vi "Zluta-Rolnicky.vi"(11 "NXT/EV3":T1) -> (3 "NXT/EV3 2":T1)   [LabVIEW 2016]
uses:
  <vilib>/NXT/Subs/LVHSConnector.ctl
  <vilib>/NXT/LegoClasses/BrickReference/BrickReference.lvclass
  <vilib>/NXT/Dual Mode Library/Display/drawText_Center.vi
  <vilib>/NXT/Dual Mode Library/Sound/PlayD.vi
  <vilib>/NXT/Dual Mode Library/Sound/PlayB.vi
  <vilib>/NXT/Dual Mode Library/Sound/PlayA.vi
  <vilib>/NXT/Dual Mode Library/Sound/PlayG.vi
  <vilib>/NXT/Dual Mode Library/Sound/PlayE.vi
  <vilib>/NXT/Dual Mode Library/Sound/PlayC.vi
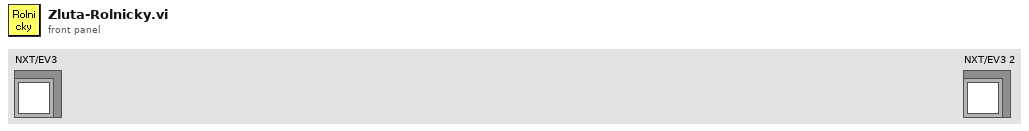
[diagram p1: front panel]
types:
  T1 = typedef "LVHSConnector.ctl" = refnum<class "BrickReference.lvclass">
diagram:
  w13 = u16 4 items=["3"=3, "4"=4, "5"=5, "6"=6, "7"=7] ("Octave")
  w14 = u16 4 items=["3"=3, "4"=4, "5"=5, "6"=6, "7"=7] ("Octave")
  w10 = u16 5 items=["3"=3, "4"=4, "5"=5, "6"=6, "7"=7] ("Octave")
  w5 = u16 5 items=["3"=3, "4"=4, "5"=5, "6"=6, "7"=7] ("Octave")
  w4 = u16 5 items=["3"=3, "4"=4, "5"=5, "6"=6, "7"=7] ("Octave")
  w20 = u16 4 items=["3"=3, "4"=4, "5"=5, "6"=6, "7"=7] ("Octave")
  w23 = u16 4 items=["3"=3, "4"=4, "5"=5, "6"=6, "7"=7] ("Octave")
  w28 = u16 4 items=["3"=3, "4"=4, "5"=5, "6"=6, "7"=7] ("Octave")
  w29 = u16 5 items=["3"=3, "4"=4, "5"=5, "6"=6, "7"=7] ("Octave")
  w38 = u16 5 items=["3"=3, "4"=4, "5"=5, "6"=6, "7"=7] ("Octave")
  w33 = u16 5 items=["3"=3, "4"=4, "5"=5, "6"=6, "7"=7] ("Octave")
  w32 = u16 5 items=["3"=3, "4"=4, "5"=5, "6"=6, "7"=7] ("Octave")
  w43 = u16 4 items=["3"=3, "4"=4, "5"=5, "6"=6, "7"=7] ("Octave")
  w44 = u16 4 items=["3"=3, "4"=4, "5"=5, "6"=6, "7"=7] ("Octave")
  w47 = u16 4 items=["3"=3, "4"=4, "5"=5, "6"=6, "7"=7] ("Octave")
  w50 = u16 5 items=["3"=3, "4"=4, "5"=5, "6"=6, "7"=7] ("Octave")
  w53 = u16 4 items=["3"=3, "4"=4, "5"=5, "6"=6, "7"=7] ("Octave")
  w62 = u16 4 items=["3"=3, "4"=4, "5"=5, "6"=6, "7"=7] ("Octave")
  w57 = u16 4 items=["3"=3, "4"=4, "5"=5, "6"=6, "7"=7] ("Octave")
  w56 = u16 4 items=["3"=3, "4"=4, "5"=5, "6"=6, "7"=7] ("Octave")
  w63 = u16 4 items=["3"=3, "4"=4, "5"=5, "6"=6, "7"=7] ("Octave")
  w68 = u16 4 items=["3"=3, "4"=4, "5"=5, "6"=6, "7"=7] ("Octave")
  w69 = u16 4 items=["3"=3, "4"=4, "5"=5, "6"=6, "7"=7] ("Octave")
  w73 = u16 5 items=["3"=3, "4"=4, "5"=5, "6"=6, "7"=7] ("Octave")
  w74 = u16 4 items=["3"=3, "4"=4, "5"=5, "6"=6, "7"=7] ("Octave")
  w78 = u16 4 items=["3"=3, "4"=4, "5"=5, "6"=6, "7"=7] ("Octave")
  w82 = u16 4 items=["3"=3, "4"=4, "5"=5, "6"=6, "7"=7] ("Octave")
  w84 = u16 4 items=["3"=3, "4"=4, "5"=5, "6"=6, "7"=7] ("Octave")
  w86 = u16 4 items=["3"=3, "4"=4, "5"=5, "6"=6, "7"=7] ("Octave")
  w91 = u16 4 items=["3"=3, "4"=4, "5"=5, "6"=6, "7"=7] ("Octave")
  w96 = u16 4 items=["3"=3, "4"=4, "5"=5, "6"=6, "7"=7] ("Octave")
  w97 = u16 5 items=["3"=3, "4"=4, "5"=5, "6"=6, "7"=7] ("Octave")
  w106 = u16 5 items=["3"=3, "4"=4, "5"=5, "6"=6, "7"=7] ("Octave")
  w101 = u16 5 items=["3"=3, "4"=4, "5"=5, "6"=6, "7"=7] ("Octave")
  w100 = u16 5 items=["3"=3, "4"=4, "5"=5, "6"=6, "7"=7] ("Octave")
  w112 = u16 4 items=["3"=3, "4"=4, "5"=5, "6"=6, "7"=7] ("Octave")
  w113 = u16 4 items=["3"=3, "4"=4, "5"=5, "6"=6, "7"=7] ("Octave")
  w116 = u16 4 items=["3"=3, "4"=4, "5"=5, "6"=6, "7"=7] ("Octave")
  w119 = u16 5 items=["3"=3, "4"=4, "5"=5, "6"=6, "7"=7] ("Octave")
  w122 = u16 4 items=["3"=3, "4"=4, "5"=5, "6"=6, "7"=7] ("Octave")
  w131 = u16 4 items=["3"=3, "4"=4, "5"=5, "6"=6, "7"=7] ("Octave")
  w126 = u16 4 items=["3"=3, "4"=4, "5"=5, "6"=6, "7"=7] ("Octave")
  w125 = u16 4 items=["3"=3, "4"=4, "5"=5, "6"=6, "7"=7] ("Octave")
  w132 = u16 4 items=["3"=3, "4"=4, "5"=5, "6"=6, "7"=7] ("Octave")
  w137 = u16 4 items=["3"=3, "4"=4, "5"=5, "6"=6, "7"=7] ("Octave")
  w138 = u16 4 items=["3"=3, "4"=4, "5"=5, "6"=6, "7"=7] ("Octave")
  w196 = u16 4 items=["3"=3, "4"=4, "5"=5, "6"=6, "7"=7] ("Octave")
  w195 = u16 4 items=["3"=3, "4"=4, "5"=5, "6"=6, "7"=7] ("Octave")
  w194 = u16 5 items=["3"=3, "4"=4, "5"=5, "6"=6, "7"=7] ("Octave")
  w193 = u16 5 items=["3"=3, "4"=4, "5"=5, "6"=6, "7"=7] ("Octave")
  w192 = u16 5 items=["3"=3, "4"=4, "5"=5, "6"=6, "7"=7] ("Octave")
  w178 = u16 5 items=["3"=3, "4"=4, "5"=5, "6"=6, "7"=7] ("Octave")
  w175 = u16 5 items=["3"=3, "4"=4, "5"=5, "6"=6, "7"=7] ("Octave")
  w174 = u16 5 items=["3"=3, "4"=4, "5"=5, "6"=6, "7"=7] ("Octave")
  w173 = u16 5 items=["3"=3, "4"=4, "5"=5, "6"=6, "7"=7] ("Octave")
  w197 = u16 4 items=["3"=3, "4"=4, "5"=5, "6"=6, "7"=7] ("Octave")
  w198 = u16 4 items=["3"=3, "4"=4, "5"=5, "6"=6, "7"=7] ("Octave")
  w199 = u16 5 items=["3"=3, "4"=4, "5"=5, "6"=6, "7"=7] ("Octave")
  w200 = u16 5 items=["3"=3, "4"=4, "5"=5, "6"=6, "7"=7] ("Octave")
  w201 = u16 5 items=["3"=3, "4"=4, "5"=5, "6"=6, "7"=7] ("Octave")
  w215 = u16 5 items=["3"=3, "4"=4, "5"=5, "6"=6, "7"=7] ("Octave")
  w218 = u16 5 items=["3"=3, "4"=4, "5"=5, "6"=6, "7"=7] ("Octave")
  w219 = u16 5 items=["3"=3, "4"=4, "5"=5, "6"=6, "7"=7] ("Octave")
  w220 = u16 5 items=["3"=3, "4"=4, "5"=5, "6"=6, "7"=7] ("Octave")
  w255 = i16 0 items=["1", "2", "3", "4", "5", "6", "7", "8", "9", "10", "11", "12"] ("Line")
  n1 = call-poly <vilib>:"PolyDisplay.vi"("Text"="\n\n\n\n\nEV3 JUK3BOX:\nRolnicky \n\n\n\n\n\n\n\n\n\n", "NXT/EV3"="NXT/EV3", "Line"=w255) -> ("NXT/EV3"=w230:T1)  [unwired: 1 in]
  n2 = call-poly <vilib>:"PolySound.vi"("Duration (500 ms)"=u16 375, "NXT/EV3"=w230) -> ("NXT/EV3"=w251:T1)  [unwired: 2 in]
  n3 = call-poly <vilib>:"PolySound.vi"("Duration (500 ms)"=u16 375, "NXT/EV3"=w251) -> ("NXT/EV3"=w247:T1)  [unwired: 2 in]
  n4 = call-poly <vilib>:"PolySound.vi"("Duration (500 ms)"=u16 375, "NXT/EV3"=w247) -> ("NXT/EV3"=w246:T1)  [unwired: 2 in]
  n5 = call-poly <vilib>:"PolySound.vi"("Duration (500 ms)"=u16 375, "NXT/EV3"=w246) -> ("NXT/EV3"=w245:T1)  [unwired: 2 in]
  n6 = call-poly <vilib>:"PolySound.vi"("Duration (500 ms)"=u16 1125, "NXT/EV3"=w245) -> ("NXT/EV3"=w242:T1)  [unwired: 2 in]
  n7 = call-poly <vilib>:"PolySound.vi"("Duration (500 ms)"=u16 375, "NXT/EV3"=w242) -> ("NXT/EV3"=w241:T1)  [unwired: 2 in]
  n8 = call-poly <vilib>:"PolySound.vi"("Duration (500 ms)"=u16 375, "NXT/EV3"=w241) -> ("NXT/EV3"=w235:T1)  [unwired: 2 in]
  n9 = call-poly <vilib>:"PolySound.vi"("Duration (500 ms)"=u16 375, "NXT/EV3"=w235) -> ("NXT/EV3"=w236:T1)  [unwired: 2 in]
  n10 = call-poly <vilib>:"PolySound.vi"("Duration (500 ms)"=u16 375, "NXT/EV3"=w236) -> ("NXT/EV3"=w240:T1)  [unwired: 2 in]
  n11 = call-poly <vilib>:"PolySound.vi"("Duration (500 ms)"=u16 375, "NXT/EV3"=w240) -> ("NXT/EV3"=w231:T1)  [unwired: 2 in]
  n12 = call-poly <vilib>:"PolySound.vi"("Duration (500 ms)"=u16 1125, "NXT/EV3"=w231) -> ("NXT/EV3"=w234:T1)  [unwired: 2 in]
  n13 = call-poly <vilib>:"PolySound.vi"("Duration (500 ms)"=u16 375, "NXT/EV3"=w234) -> ("NXT/EV3"=w202:T1)  [unwired: 2 in]
  n14 = call-poly <vilib>:"PolySound.vi"("Duration (500 ms)"=u16 375, "NXT/EV3"=w202) -> ("NXT/EV3"=w223:T1)  [unwired: 2 in]
  n15 = call-poly <vilib>:"PolySound.vi"("Duration (500 ms)"=u16 375, "NXT/EV3"=w223, "Octave"=w220) -> ("NXT/EV3"=w227:T1)  [unwired: 1 in]
  n16 = call-poly <vilib>:"PolySound.vi"("Duration (500 ms)"=u16 375, "NXT/EV3"=w227) -> ("NXT/EV3"=w228:T1)  [unwired: 2 in]
  n17 = call-poly <vilib>:"PolySound.vi"("Duration (500 ms)"=u16 375, "NXT/EV3"=w228) -> ("NXT/EV3"=w229:T1)  [unwired: 2 in]
  n18 = call-poly <vilib>:"PolySound.vi"("Duration (500 ms)"=u16 375, "NXT/EV3"=w229, "Octave"=w219) -> ("NXT/EV3"=w214:T1)  [unwired: 1 in]
  n19 = call-poly <vilib>:"PolySound.vi"("Duration (500 ms)"=u16 375, "NXT/EV3"=w214, "Octave"=w218) -> ("NXT/EV3"=w213:T1)  [unwired: 1 in]
  n20 = call-poly <vilib>:"PolySound.vi"("Duration (500 ms)"=u16 750, "NXT/EV3"=w213, "Octave"=w215) -> ("NXT/EV3"=w207:T1)  [unwired: 1 in]
  n21 = call-poly <vilib>:"PolySound.vi"("Duration (500 ms)"=u16 375, "NXT/EV3"=w207, "Octave"=w201) -> ("NXT/EV3"=w206:T1)  [unwired: 1 in]
  n22 = call-poly <vilib>:"PolySound.vi"("Duration (500 ms)"=u16 375, "NXT/EV3"=w206, "Octave"=w200) -> ("NXT/EV3"=w205:T1)  [unwired: 1 in]
  n23 = call-poly <vilib>:"PolySound.vi"("Duration (500 ms)"=u16 375, "NXT/EV3"=w205, "Octave"=w199) -> ("NXT/EV3"=w204:T1)  [unwired: 1 in]
  n24 = call-poly <vilib>:"PolySound.vi"("Duration (500 ms)"=u16 375, "NXT/EV3"=w204, "Octave"=w198) -> ("NXT/EV3"=w203:T1)  [unwired: 1 in]
  n25 = call-poly <vilib>:"PolySound.vi"("Duration (500 ms)"=u16 1500, "NXT/EV3"=w203, "Octave"=w197) -> ("NXT/EV3"=w140:T1)  [unwired: 1 in]
  n26 = call-poly <vilib>:"PolySound.vi"("Duration (500 ms)"=u16 375, "NXT/EV3"=w140) -> ("NXT/EV3"=w143:T1)  [unwired: 2 in]
  n27 = call-poly <vilib>:"PolySound.vi"("Duration (500 ms)"=u16 375, "NXT/EV3"=w143) -> ("NXT/EV3"=w147:T1)  [unwired: 2 in]
  n28 = call-poly <vilib>:"PolySound.vi"("Duration (500 ms)"=u16 375, "NXT/EV3"=w147) -> ("NXT/EV3"=w148:T1)  [unwired: 2 in]
  n29 = call-poly <vilib>:"PolySound.vi"("Duration (500 ms)"=u16 375, "NXT/EV3"=w148) -> ("NXT/EV3"=w149:T1)  [unwired: 2 in]
  n30 = call-poly <vilib>:"PolySound.vi"("Duration (500 ms)"=u16 1125, "NXT/EV3"=w149) -> ("NXT/EV3"=w152:T1)  [unwired: 2 in]
  n31 = call-poly <vilib>:"PolySound.vi"("Duration (500 ms)"=u16 375, "NXT/EV3"=w152) -> ("NXT/EV3"=w153:T1)  [unwired: 2 in]
  n32 = call-poly <vilib>:"PolySound.vi"("Duration (500 ms)"=u16 375, "NXT/EV3"=w153) -> ("NXT/EV3"=w159:T1)  [unwired: 2 in]
  n33 = call-poly <vilib>:"PolySound.vi"("Duration (500 ms)"=u16 375, "NXT/EV3"=w159) -> ("NXT/EV3"=w158:T1)  [unwired: 2 in]
  n34 = call-poly <vilib>:"PolySound.vi"("Duration (500 ms)"=u16 375, "NXT/EV3"=w158) -> ("NXT/EV3"=w154:T1)  [unwired: 2 in]
  n35 = call-poly <vilib>:"PolySound.vi"("Duration (500 ms)"=u16 375, "NXT/EV3"=w154) -> ("NXT/EV3"=w163:T1)  [unwired: 2 in]
  n36 = call-poly <vilib>:"PolySound.vi"("Duration (500 ms)"=u16 1125, "NXT/EV3"=w163) -> ("NXT/EV3"=w160:T1)  [unwired: 2 in]
  n37 = call-poly <vilib>:"PolySound.vi"("Duration (500 ms)"=u16 375, "NXT/EV3"=w160) -> ("NXT/EV3"=w191:T1)  [unwired: 2 in]
  n38 = call-poly <vilib>:"PolySound.vi"("Duration (500 ms)"=u16 375, "NXT/EV3"=w191) -> ("NXT/EV3"=w170:T1)  [unwired: 2 in]
  n39 = call-poly <vilib>:"PolySound.vi"("Duration (500 ms)"=u16 375, "NXT/EV3"=w170, "Octave"=w173) -> ("NXT/EV3"=w166:T1)  [unwired: 1 in]
  n40 = call-poly <vilib>:"PolySound.vi"("Duration (500 ms)"=u16 375, "NXT/EV3"=w166) -> ("NXT/EV3"=w165:T1)  [unwired: 2 in]
  n41 = call-poly <vilib>:"PolySound.vi"("Duration (500 ms)"=u16 375, "NXT/EV3"=w165) -> ("NXT/EV3"=w164:T1)  [unwired: 2 in]
  n42 = call-poly <vilib>:"PolySound.vi"("Duration (500 ms)"=u16 375, "NXT/EV3"=w164, "Octave"=w174) -> ("NXT/EV3"=w179:T1)  [unwired: 1 in]
  n43 = call-poly <vilib>:"PolySound.vi"("Duration (500 ms)"=u16 375, "NXT/EV3"=w179, "Octave"=w175) -> ("NXT/EV3"=w180:T1)  [unwired: 1 in]
  n44 = call-poly <vilib>:"PolySound.vi"("Duration (500 ms)"=u16 750, "NXT/EV3"=w180, "Octave"=w178) -> ("NXT/EV3"=w186:T1)  [unwired: 1 in]
  n45 = call-poly <vilib>:"PolySound.vi"("Duration (500 ms)"=u16 375, "NXT/EV3"=w186, "Octave"=w192) -> ("NXT/EV3"=w187:T1)  [unwired: 1 in]
  n46 = call-poly <vilib>:"PolySound.vi"("Duration (500 ms)"=u16 375, "NXT/EV3"=w187, "Octave"=w193) -> ("NXT/EV3"=w188:T1)  [unwired: 1 in]
  n47 = call-poly <vilib>:"PolySound.vi"("Duration (500 ms)"=u16 375, "NXT/EV3"=w188, "Octave"=w194) -> ("NXT/EV3"=w189:T1)  [unwired: 1 in]
  n48 = call-poly <vilib>:"PolySound.vi"("Duration (500 ms)"=u16 375, "NXT/EV3"=w189, "Octave"=w195) -> ("NXT/EV3"=w190:T1)  [unwired: 1 in]
  n49 = call-poly <vilib>:"PolySound.vi"("Duration (500 ms)"=u16 1500, "NXT/EV3"=w190, "Octave"=w196) -> ("NXT/EV3"=w107:T1)  [unwired: 1 in]
  n50 = call-poly <vilib>:"PolySound.vi"("Duration (500 ms)"=u16 375, "NXT/EV3"=w107, "Octave"=w138) -> ("NXT/EV3"=w134:T1)  [unwired: 1 in]
  n51 = call-poly <vilib>:"PolySound.vi"("Duration (500 ms)"=u16 375, "NXT/EV3"=w134, "Octave"=w137) -> ("NXT/EV3"=w133:T1)  [unwired: 1 in]
  n52 = call-poly <vilib>:"PolySound.vi"("Duration (500 ms)"=u16 750, "NXT/EV3"=w133, "Octave"=w132) -> ("NXT/EV3"=w123:T1)  [unwired: 1 in]
  n53 = call-poly <vilib>:"PolySound.vi"("Duration (500 ms)"=u16 375, "NXT/EV3"=w123, "Octave"=w125) -> ("NXT/EV3"=w129:T1)  [unwired: 1 in]
  n54 = call-poly <vilib>:"PolySound.vi"("Duration (500 ms)"=u16 375, "NXT/EV3"=w129, "Octave"=w126) -> ("NXT/EV3"=w130:T1)  [unwired: 1 in]
  n55 = call-poly <vilib>:"PolySound.vi"("Duration (500 ms)"=u16 750, "NXT/EV3"=w130, "Octave"=w131) -> ("NXT/EV3"=w117:T1)  [unwired: 1 in]
  n56 = call-poly <vilib>:"PolySound.vi"("Duration (500 ms)"=u16 375, "NXT/EV3"=w117, "Octave"=w122) -> ("NXT/EV3"=w118:T1)  [unwired: 1 in]
  n57 = call-poly <vilib>:"PolySound.vi"("Duration (500 ms)"=u16 375, "NXT/EV3"=w118, "Octave"=w119) -> ("NXT/EV3"=w108:T1)  [unwired: 1 in]
  n58 = call-poly <vilib>:"PolySound.vi"("Duration (500 ms)"=u16 562, "NXT/EV3"=w108, "Octave"=w116) -> ("NXT/EV3"=w110:T1)  [unwired: 1 in]
  n59 = call-poly <vilib>:"PolySound.vi"("Duration (500 ms)"=u16 188, "NXT/EV3"=w110, "Octave"=w113) -> ("NXT/EV3"=w109:T1)  [unwired: 1 in]
  n60 = call-poly <vilib>:"PolySound.vi"("Duration (500 ms)"=u16 1500, "NXT/EV3"=w109, "Octave"=w112) -> ("NXT/EV3"=w89:T1)  [unwired: 1 in]
  n61 = call-poly <vilib>:"PolySound.vi"("Duration (500 ms)"=u16 375, "NXT/EV3"=w89, "Octave"=w100) -> ("NXT/EV3"=w104:T1)  [unwired: 1 in]
  n62 = call-poly <vilib>:"PolySound.vi"("Duration (500 ms)"=u16 375, "NXT/EV3"=w104, "Octave"=w101) -> ("NXT/EV3"=w105:T1)  [unwired: 1 in]
  n63 = call-poly <vilib>:"PolySound.vi"("Duration (500 ms)"=u16 750, "NXT/EV3"=w105, "Octave"=w106) -> ("NXT/EV3"=w90:T1)  [unwired: 1 in]
  n64 = call-poly <vilib>:"PolySound.vi"("Duration (500 ms)"=u16 375, "NXT/EV3"=w90, "Octave"=w97) -> ("NXT/EV3"=w93:T1)  [unwired: 1 in]
  n65 = call-poly <vilib>:"PolySound.vi"("Duration (500 ms)"=u16 375, "NXT/EV3"=w93, "Octave"=w96) -> ("NXT/EV3"=w92:T1)  [unwired: 1 in]
  n66 = call-poly <vilib>:"PolySound.vi"("Duration (500 ms)"=u16 750, "NXT/EV3"=w92, "Octave"=w91) -> ("NXT/EV3"=w83:T1)  [unwired: 1 in]
  n67 = call-poly <vilib>:"PolySound.vi"("Duration (500 ms)"=u16 375, "NXT/EV3"=w83, "Octave"=w86) -> ("NXT/EV3"=w88:T1)  [unwired: 1 in]
  n68 = call-poly <vilib>:"PolySound.vi"("Duration (500 ms)"=u16 375, "NXT/EV3"=w88, "Octave"=w84) -> ("NXT/EV3"=w80:T1)  [unwired: 1 in]
  n69 = call-poly <vilib>:"PolySound.vi"("Duration (500 ms)"=u16 375, "NXT/EV3"=w80, "Octave"=w82) -> ("NXT/EV3"=w77:T1)  [unwired: 1 in]
  n70 = call-poly <vilib>:"PolySound.vi"("Duration (500 ms)"=u16 375, "NXT/EV3"=w77, "Octave"=w78) -> ("NXT/EV3"=w75:T1)  [unwired: 1 in]
  n71 = call-poly <vilib>:"PolySound.vi"("Duration (500 ms)"=u16 750, "NXT/EV3"=w75, "Octave"=w74) -> ("NXT/EV3"=w71:T1)  [unwired: 1 in]
  n72 = call-poly <vilib>:"PolySound.vi"("Duration (500 ms)"=u16 750, "NXT/EV3"=w71, "Octave"=w73) -> ("NXT/EV3"=w17:T1)  [unwired: 1 in]
  n73 = call-poly <vilib>:"PolySound.vi"("Duration (500 ms)"=u16 375, "NXT/EV3"=w17, "Octave"=w69) -> ("NXT/EV3"=w65:T1)  [unwired: 1 in]
  n74 = call-poly <vilib>:"PolySound.vi"("Duration (500 ms)"=u16 375, "NXT/EV3"=w65, "Octave"=w68) -> ("NXT/EV3"=w64:T1)  [unwired: 1 in]
  n75 = call-poly <vilib>:"PolySound.vi"("Duration (500 ms)"=u16 750, "NXT/EV3"=w64, "Octave"=w63) -> ("NXT/EV3"=w54:T1)  [unwired: 1 in]
  n76 = call-poly <vilib>:"PolySound.vi"("Duration (500 ms)"=u16 375, "NXT/EV3"=w54, "Octave"=w56) -> ("NXT/EV3"=w60:T1)  [unwired: 1 in]
  n77 = call-poly <vilib>:"PolySound.vi"("Duration (500 ms)"=u16 375, "NXT/EV3"=w60, "Octave"=w57) -> ("NXT/EV3"=w61:T1)  [unwired: 1 in]
  n78 = call-poly <vilib>:"PolySound.vi"("Duration (500 ms)"=u16 750, "NXT/EV3"=w61, "Octave"=w62) -> ("NXT/EV3"=w48:T1)  [unwired: 1 in]
  n79 = call-poly <vilib>:"PolySound.vi"("Duration (500 ms)"=u16 375, "NXT/EV3"=w48, "Octave"=w53) -> ("NXT/EV3"=w49:T1)  [unwired: 1 in]
  n80 = call-poly <vilib>:"PolySound.vi"("Duration (500 ms)"=u16 375, "NXT/EV3"=w49, "Octave"=w50) -> ("NXT/EV3"=w39:T1)  [unwired: 1 in]
  n81 = call-poly <vilib>:"PolySound.vi"("Duration (500 ms)"=u16 562, "NXT/EV3"=w39, "Octave"=w47) -> ("NXT/EV3"=w41:T1)  [unwired: 1 in]
  n82 = call-poly <vilib>:"PolySound.vi"("Duration (500 ms)"=u16 188, "NXT/EV3"=w41, "Octave"=w44) -> ("NXT/EV3"=w40:T1)  [unwired: 1 in]
  n83 = call-poly <vilib>:"PolySound.vi"("Duration (500 ms)"=u16 1500, "NXT/EV3"=w40, "Octave"=w43) -> ("NXT/EV3"=w21:T1)  [unwired: 1 in]
  n84 = call-poly <vilib>:"PolySound.vi"("Duration (500 ms)"=u16 375, "NXT/EV3"=w21, "Octave"=w32) -> ("NXT/EV3"=w36:T1)  [unwired: 1 in]
  n85 = call-poly <vilib>:"PolySound.vi"("Duration (500 ms)"=u16 375, "NXT/EV3"=w36, "Octave"=w33) -> ("NXT/EV3"=w37:T1)  [unwired: 1 in]
  n86 = call-poly <vilib>:"PolySound.vi"("Duration (500 ms)"=u16 750, "NXT/EV3"=w37, "Octave"=w38) -> ("NXT/EV3"=w22:T1)  [unwired: 1 in]
  n87 = call-poly <vilib>:"PolySound.vi"("Duration (500 ms)"=u16 375, "NXT/EV3"=w22, "Octave"=w29) -> ("NXT/EV3"=w25:T1)  [unwired: 1 in]
  n88 = call-poly <vilib>:"PolySound.vi"("Duration (500 ms)"=u16 375, "NXT/EV3"=w25, "Octave"=w28) -> ("NXT/EV3"=w24:T1)  [unwired: 1 in]
  n89 = call-poly <vilib>:"PolySound.vi"("Duration (500 ms)"=u16 750, "NXT/EV3"=w24, "Octave"=w23) -> ("NXT/EV3"=w18:T1)  [unwired: 1 in]
  n90 = call-poly <vilib>:"PolySound.vi"("Duration (500 ms)"=u16 375, "NXT/EV3"=w18, "Octave"=w20) -> ("NXT/EV3"=w2:T1)  [unwired: 1 in]
  n91 = call-poly <vilib>:"PolySound.vi"("Duration (500 ms)"=u16 375, "NXT/EV3"=w2, "Octave"=w4) -> ("NXT/EV3"=w8:T1)  [unwired: 1 in]
  n92 = call-poly <vilib>:"PolySound.vi"("Duration (500 ms)"=u16 375, "NXT/EV3"=w8, "Octave"=w5) -> ("NXT/EV3"=w9:T1)  [unwired: 1 in]
  n93 = call-poly <vilib>:"PolySound.vi"("Duration (500 ms)"=u16 750, "NXT/EV3"=w9, "Octave"=w10) -> ("NXT/EV3"=w16:T1)  [unwired: 1 in]
  n94 = call-poly <vilib>:"PolySound.vi"("Duration (500 ms)"=u16 375, "NXT/EV3"=w16, "Octave"=w14) -> ("NXT/EV3"=w11:T1)  [unwired: 1 in]
  n95 = call-poly <vilib>:"PolySound.vi"("Duration (500 ms)"=u16 850, "NXT/EV3"=w11, "Octave"=w13) -> ("NXT/EV3"=→"NXT/EV3 2":T1)  [unwired: 1 in]
